vi "Save User Devices.vi"(8 "error in (no error)":errorcluster, 11 "picoG in":refnum<class "picoG.lvclass">) -> (0 "error out":errorcluster, 3 "picoG out":refnum<class "picoG.lvclass">)   [LabVIEW 2020, in "PicoG-App.lvlib" / "picoG.lvclass"]
uses:
  picoG.lvclass
  picoG.lvclass/picoG.ctl
  <vilib>/Utility/config.llb/Write Key (I32).vi
  PicoG-App.lvlib
  <vilib>/Utility/config.llb/NI_LVConfig.lvlib
  DeviceListPanel/DeviceListPanel.lvclass
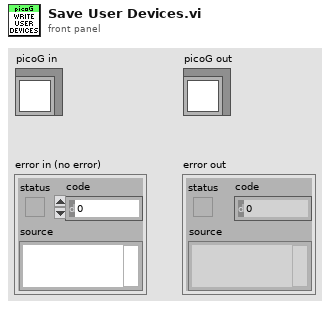
[diagram p1: front panel]
types:
  T1 = typedef "PicoG-App.lvlib/Paths.ctl" = cluster{"User picoG":path, "System picoG":path, "User Config":path, "System Config":path}
  T2 = typedef "NI_LVConfig.lvlib/Config Data RefNum.ctl" = refnum<k1>
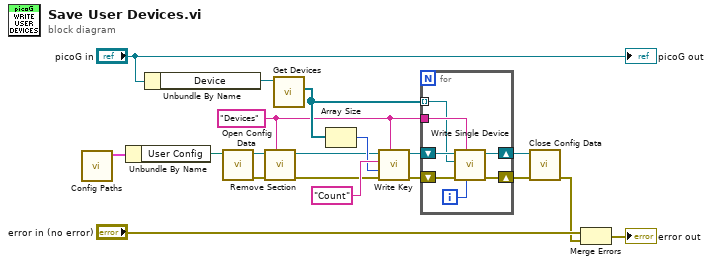
[diagram p0: block diagram]
diagram:
  w1 = "Devices" ("section")
  n1 = call "Config Paths.vi"() -> ("Paths"=w18:T1)  [unwired: 8 in, 3 out]
  n2 = Unbundle By Name(w18) -> ("User Config"=w17:path)
  n3 = Unbundle By Name("picoG in") -> ("Device"=w13:refnum<class "DeviceListPanel.lvclass">)
  n4 = call <vilib>:"Open Config Data.vi"("configuration file path"=w17) -> ("error out"=w15:errorcluster, "refnum"=w16:T2)  [unwired: 8 in, 1 out]
  n5 = call <vilib>:"Remove Section.vi"("section"=w1, "error in (no error)"=w15, "refnum"=w16) -> ("error out"=w10:errorcluster, "refnum out"=w9:T2)  [unwired: 6 in, 1 out]
  n6 = call "Get Devices.vi"("DeviceListPanel in"=w13) -> ("Devices"=w6:refnum<class "Device.lvclass">[])  [unwired: 8 in, 2 out]
  n7 = Array Size(array=w6) -> (size(s)=w11:i32)
  n8 = call-poly <vilib>:"Write Key.vi"("section"=w1, "error in (no error)"=w10, "value"=w11, "key"="Count", "refnum"=w9) -> ("error out"=w8:errorcluster, "refnum out"=w7:T2)  [unwired: 4 in, 1 out]
  n9 = for {
    shift-right: [w21] -> w4
    shift-left: w8 -> [w25]
    shift-right: [w20] -> w5
    shift-left: w7 -> [w26]
    tunnel: w1 -> [w24]
    tunnel: w6 -> [w23] mode=indexing
    i -> [w22]
    n10 = call "Write Single Device.vi"("Index"=w22, "Section"=w24, "error in (no error)"=w25, "Device"=w23, "refnum"=w26) -> ("error out"=w21:errorcluster, "refnum out"=w20:T2)  [unwired: 5 in]
  }
  n11 = call <vilib>:"Close Config Data.vi"("error in (no error)"=w4, "refnum"=w5) -> ("error out"=w2:errorcluster)  [unwired: 8 in, 1 out]
  n12 = Merge Errors("error in (no error)", w2) -> (→"error out":errorcluster)
  "picoG out" <- "picoG in"
